vi "ODX_Read Flash Data and SA2.vi"(8 "error in":errorcluster, 11 "ODX File Path":path) -> (0 "error out":errorcluster, 1 "Download Parameter":T1, 2 "SA2 Operator":T2[](array[typedef]) {"Wert" format="%.0x"}, 3 "Flash Data Array":u8[](array[numeric]))   [LabVIEW 2018]
uses:
  Typedefs/Diagnose_SA2_Rechnenbefehl.ctl
  Typedefs/Diagnose_SA2_Operation_ENUM.ctl
  <vilib>/regexp/Match Regular Expression.xnode
panel:
  out "Block Size":u8[](array[numeric]) format="%.0x"
  out "Start Adress":u8[](array[numeric]) format="%.0x"
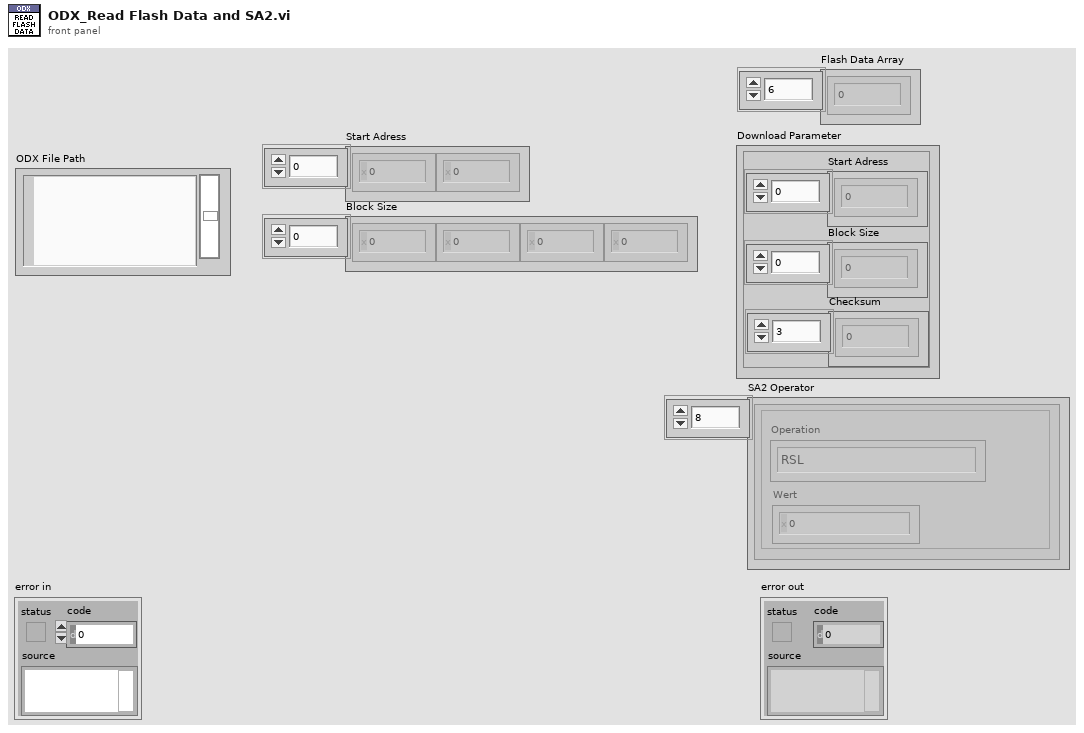
[diagram p1: front panel]
types:
  T1 = cluster{"Start Adress":u8[], "Block Size":u8[], "Checksum":u8[]}
  T2 = typedef "Diagnose_SA2_Rechnenbefehl.ctl" = cluster{"Operation":T3, "Wert":u32}
  T3 = typedef "Diagnose_SA2_Operation_ENUM.ctl" = enum16{"RSL", "RSR", "ADD", "SUB", "EOR", "Durchläufe", "NEXT", "BCC", "BRA", "Fertig"}
  T4 = enum16{"open", "replace", "create", "open or create", "replace or create", "replace or create with confirmation"}
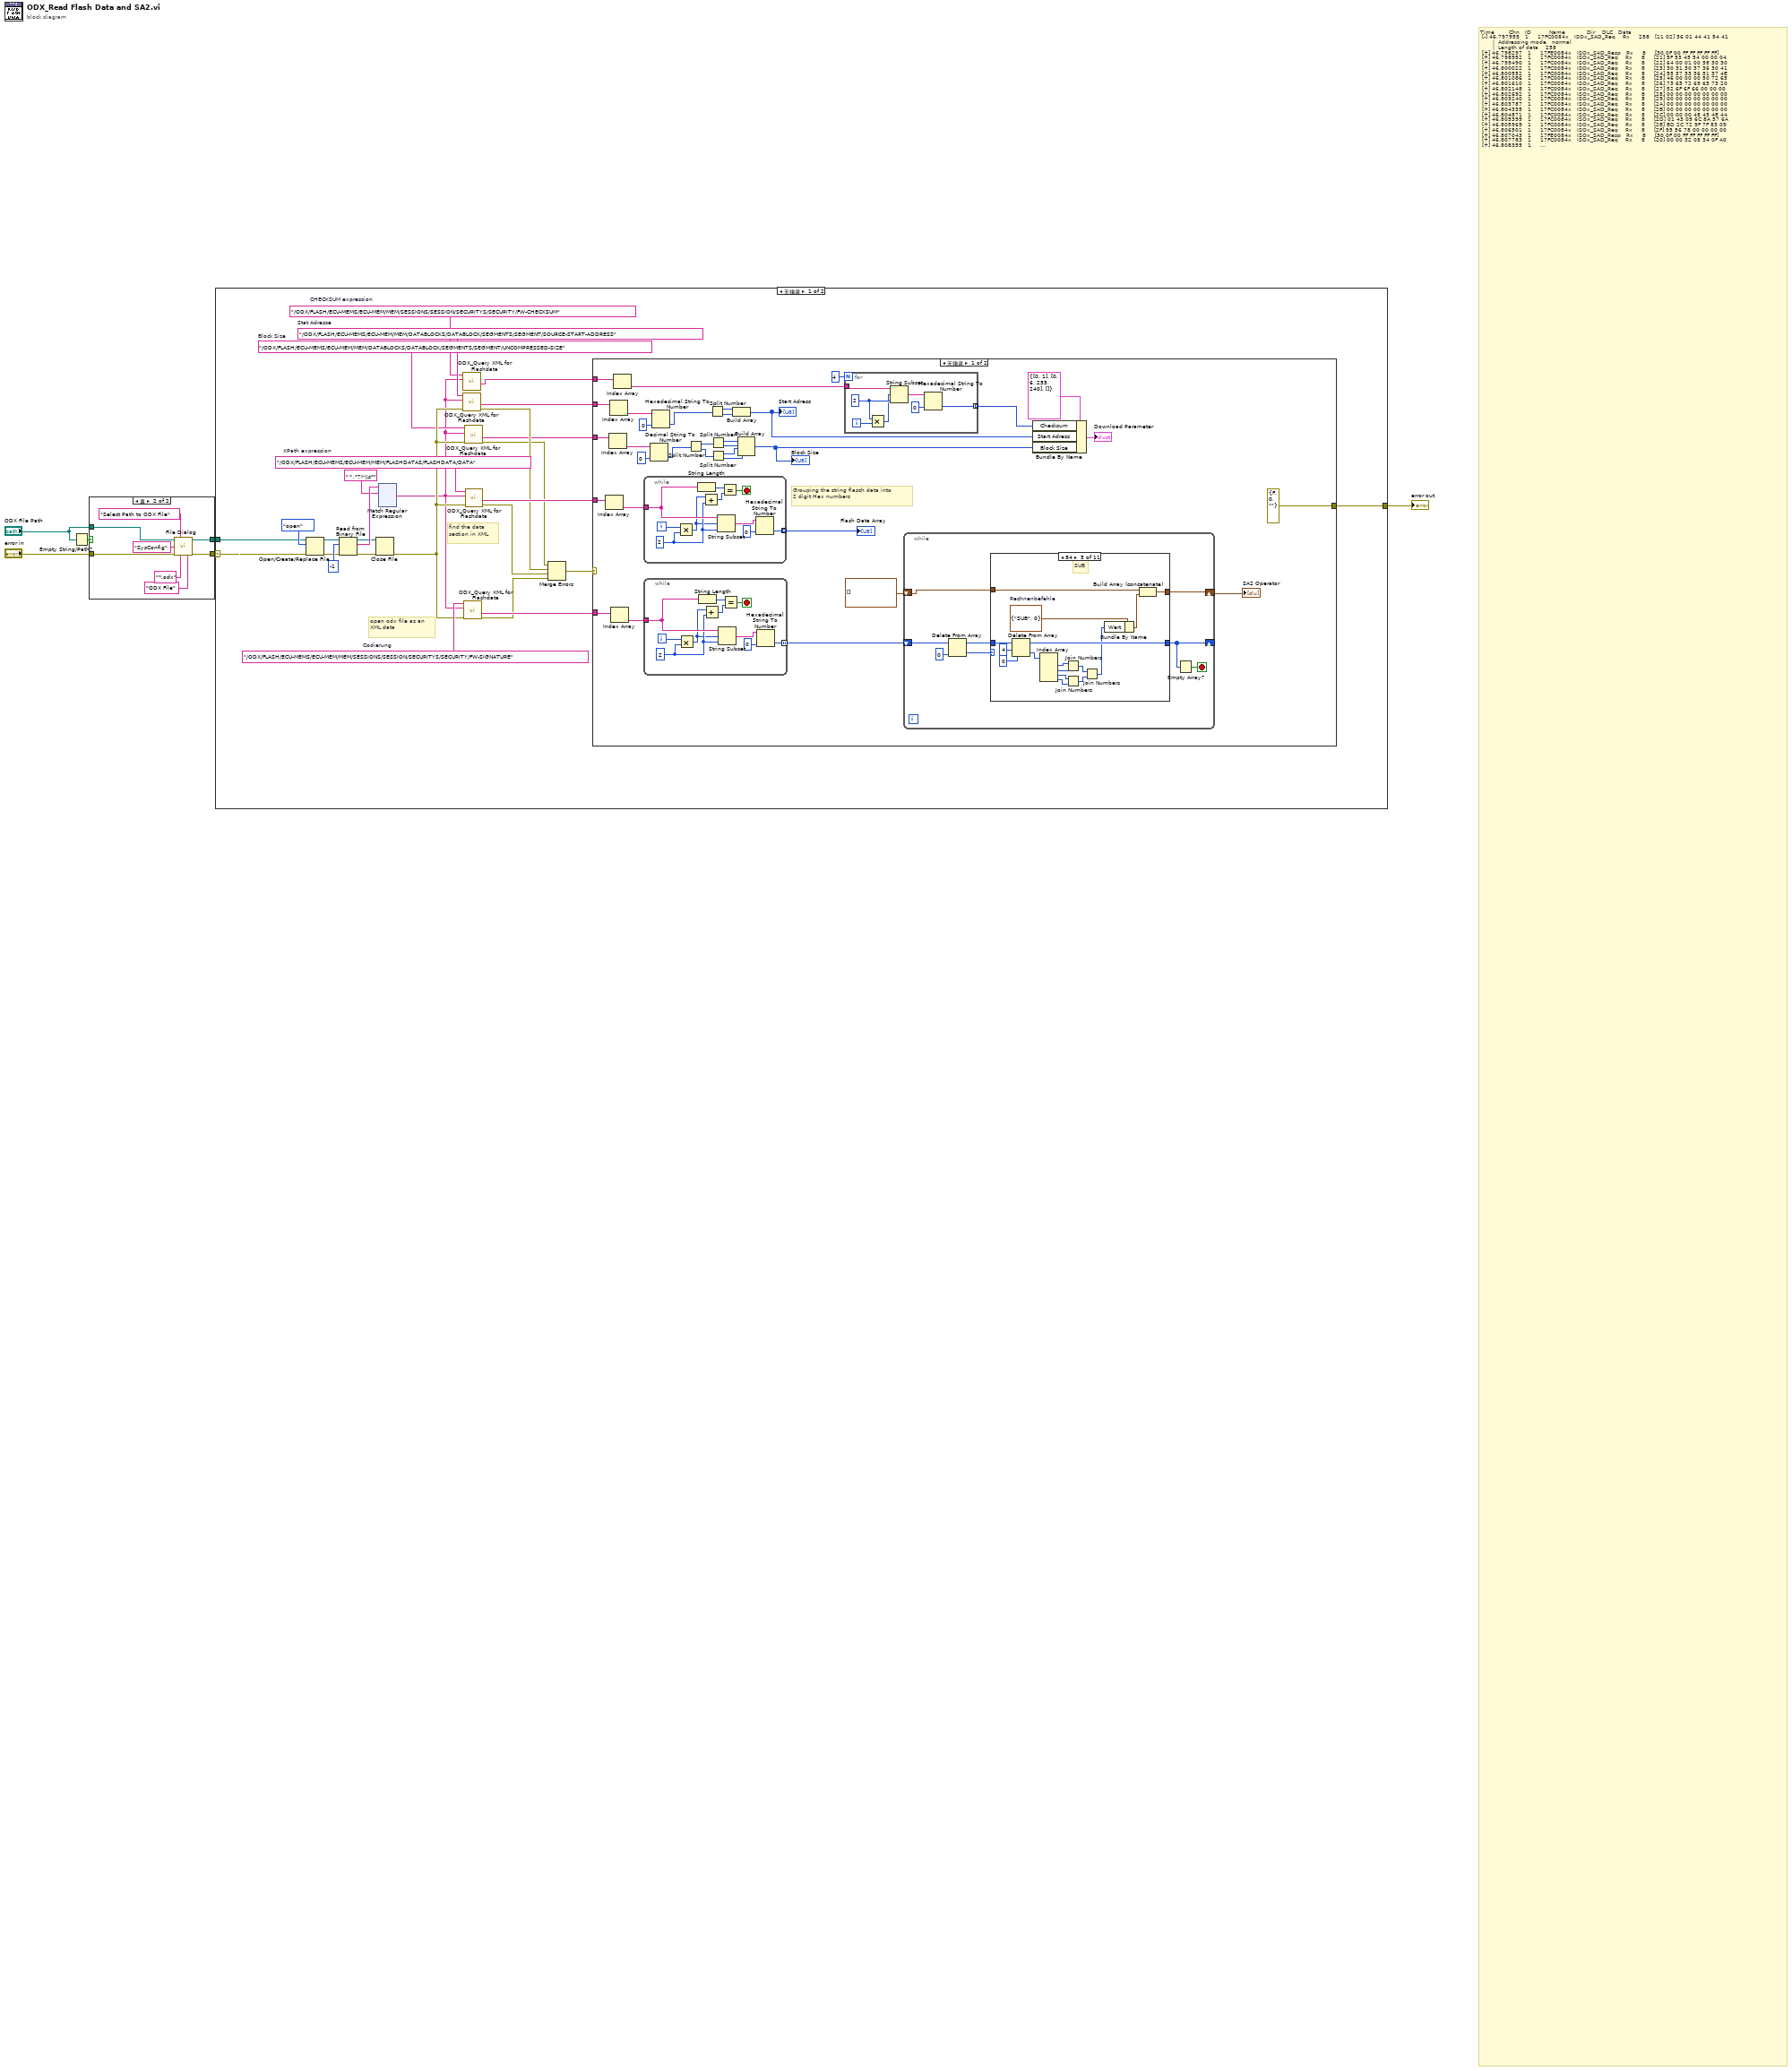
[diagram p0: block diagram]
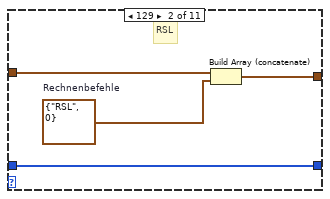
[diagram p3: hidden frame]
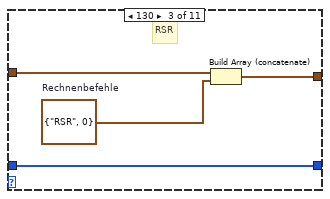
[diagram p4: hidden frame]
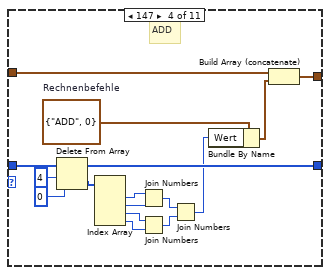
[diagram p5: hidden frame]
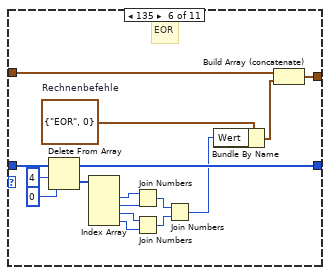
[diagram p6: hidden frame]
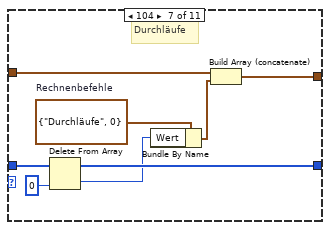
[diagram p7: hidden frame]
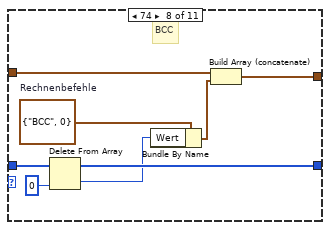
[diagram p8: hidden frame]
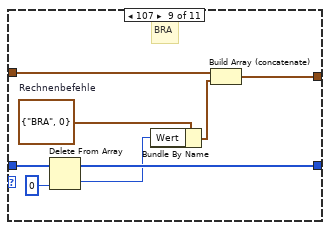
[diagram p9: hidden frame]
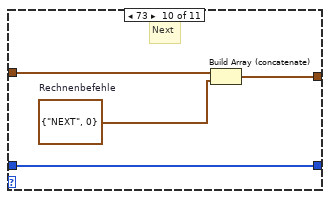
[diagram p10: hidden frame]
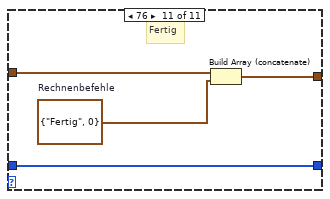
[diagram p11: hidden frame]
diagram:
  # "Time        Chn   ID          Name            Dir    DLC   Data                          \n [-] 46.797955   1     17FC0084x   ISOx_SAD_Req    Rx     258   [11 02] 36 01 44 41 54 41     \n       |  Addressing mode   normal      \n       |  Length of data    258         \n [+] 46.798297   1     17FE0084x   ISOx_SAD_Resp   Rx     8     [30 0F 00 FF FF FF FF FF]     \n [+] 46.798952   1     17FC0084x   ISOx_SAD_Req    Rx     8     [21] 5F 53 45 54 00 00 04     \n [+] 46.799490   1     17FC0084x   ISOx_SAD_Req    Rx     8     [22] 64 00 01 00 58 30 30     \n [+] 46.800022   1     17FC0084x   ISOx_SAD_Req    Rx     8     [23] 30 31 30 37 36 30 41     \n [+] 46.800552   1     17FC0084x   ISOx_SAD_Req    Rx     8     [24] 55 37 33 36 51 37 4E     \n [+] 46.801086   1     17FC0084x   ISOx_SAD_Req    Rx     8     [25] 46 00 00 00 50 72 65     \n [+] 46.801610   1     17FC0084x   ISOx_SAD_Req    Rx     8     [26] 73 65 72 69 65 73 20     \n [+] 46.802148   1     17FC0084x   ISOx_SAD_Req    Rx     8     [27] 52 6F 6F 66 00 00 00     \n [+] 46.802692   1     17FC0084x   ISOx_SAD_Req    Rx     8     [28] 00 00 00 00 00 00 00     \n [+] 46.803240   1     17FC0084x   ISOx_SAD_Req    Rx     8     [29] 00 00 00 00 00 00 00     \n [+] 46.803787   1     17FC0084x   ISOx_SAD_Req    Rx     8     [2A] 00 00 00 00 00 00 00     \n [+] 46.804335   1     17FC0084x   ISOx_SAD_Req    Rx     8     [2B] 00 00 00 00 00 00 00     \n [+] 46.804871   1     17FC0084x   ISOx_SAD_Req    Rx     8     [2C] 00 00 00 48 45 4E 44     \n [+] 46.805399   1     17FC0084x   ISOx_SAD_Req    Rx     8     [2D] 01 43 09 6C 8A 57 6A     \n [+] 46.805969   1     17FC0084x   ISOx_SAD_Req    Rx     8     [2E] BD 2C 72 9F 7F 83 09     \n [+] 46.806501   1     17FC0084x   ISOx_SAD_Req    Rx     8     [2F] 95 56 78 00 00 00 00     \n [+] 46.807043   1     17FE0084x   ISOx_SAD_Resp   Rx     8     [30 0F 00 FF FF FF FF FF]     \n [+] 46.807783   1     17FC0084x   ISOx_SAD_Req    Rx     8     [20] 00 00 32 08 34 0F A0     \n [+] 46.808355   1     17FC0084x   ISOx_SAD_Req    Rx     8     [21] 00 14 00 14 46 50 17     \n [+] 46.808930   1     17FC0084x   ISOx_SAD_Req    Rx     8     [22] 70 2E E0 1F 40 4E 20     \n [+] 46.809470   1     17FC0084x   ISOx_SAD_Req    Rx     8     [23] 1A F4 00 28 01 F4 01     \n [+] 46.810010   1     17FC0084x   ISOx_SAD_Req    Rx     8     [24] F4 00 02 00 32 00 19     \n [+] 46.810550   1     17FC0084x   ISOx_SAD_Req    Rx     8     [25] 00 96 00 32 00 00 00     \n [+] 46.811090   1     17FC0084x   ISOx_SAD_Req    Rx     8     [26] 32 00 64 00 00 00 32     \n [+] 46.811666   1     17FC0084x   ISOx_SAD_Req    Rx     8     [27] 00 64 00 50 00 50 32     \n [+] 46.812248   1     17FC0084x   ISOx_SAD_Req    Rx     8     [28] C8 01 90 07 D0 46 50     \n [+] 46.812780   1     17FC0084x   ISOx_SAD_Req    Rx     8     [29] 46 50 07 D0 6C CD 07     \n [+] 46.813316   1     17FC0084x   ISOx_SAD_Req    Rx     8     [2A] D0 1B 58 07 D0 60 00     \n [+] 46.813854   1     17FC0084x   ISOx_SAD_Req    Rx     8     [2B] 20 00 21 34 01 90 01     \n [+] 46.814389   1     17FC0084x   ISOx_SAD_Req    Rx     8     [2C] 90 01 90 01 90 01 90     \n [+] 46.814921   1     17FC0084x   ISOx_SAD_Req    Rx     8     [2D] 00 C8 5D C0 00 32 00     \n [+] 46.815459   1     17FC0084x   ISOx_SAD_Req    Rx     8     [2E] 00 01 36 06 40 00 B9     \n [+] 46.815997   1     17FE0084x   ISOx_SAD_Resp   Rx     8     [30 0F 00 FF FF FF FF FF]     \n [+] 46.816819   1     17FC0084x   ISOx_SAD_Req    Rx     8     [2F] 00 C8 00 E6 03 E8 00     \n [+] 46.817355   1     17FC0084x   ISOx_SAD_Req    Rx     8     [20] 32 00 23 00 DC 00 0A     \n [+] 46.817931   1     17FC0084x   ISOx_SAD_Req    Rx     8     [21] 00 48 1B 58 42 68 00     \n [+] 46.818466   1     17FC0084x   ISOx_SAD_Req    Rx     8     [22] C8 3E 80 3A 98 01 F4     \n [+] 46.818998   1     17FC0084x   ISOx_SAD_Req    Rx     8     [23] 2C EC 01 F4 1D 4C 03     \n [+] 46.819534   1     17FC0084x   ISOx_SAD_Req    Rx     8     [24] E8 21 34 1A 2C 02 0F     \n [+] 46.821168   1     17FE0084x   ISOx_SAD_Resp   Rx     2     [02] 76 01 [FF FF FF FF FF]   \n\n#Ende vom Block 1 (37 Messages) & Start vom Block2 (37 Messages)# \n\n[-] 46.840058   1     17FC0084x   ISOx_SAD_Req    Rx     258   [11 02] 36 02 5F 00 01 02     \n       |  Addressing mode   normal      \n       |  Length of data    258         \n [+] 46.840600   1     17FE0084x   ISOx_SAD_Resp   Rx     8     [30 0F 00 FF FF FF FF FF]     \n [+] 46.841412   1     17FC0084x   ISOx_SAD_Req    Rx     8     [21] 03 04 00 01 02 03 04     \n [+] 46.841994   1     17FC0084x   ISOx_SAD_Req    Rx     8     [22] 00 01 02 03 04 06 18     \n [+] 46.842530   1     17FC0084x   ISOx_SAD_Req    Rx     8     [23] 0A 20 1C 08 01 00 28     \n [+] 46.843066   1     17FC0084x   ISOx_SAD_Req    Rx     8     [24] 08 08 03 A0 20 C8 05     \n [+] 46.843603   1     17FC0084x   ISOx_SAD_Req    Rx     8     [25] B4 AA 05 A0 00 04 04     \n [+] 46.844129   1     17FC0084x   ISOx_SAD_Req    Rx     8     [26] 14 04 09 09 14 F6 38     \n [+] 46.844669   1     17FC0084x   ISOx_SAD_Req    Rx     8     [27] 00 00 00 01 57 C0 00     \n [+] 46.845209   1     17FC0084x   ISOx_SAD_Req    Rx     8     [28] 32 00 28 FF D8 00 14     \n [+] 46.845747   1     17FC0084x   ISOx_SAD_Req    Rx     8     [29] 07 92 00 32 00 32 01     \n [+] 46.846283   1     17FC0084x   ISOx_SAD_Req    Rx     8     [2A] 90 01 90 00 2D D8 D8     \n [+] 46.846823   1     17FC0084x   ISOx_SAD_Req    Rx     8     [2B] FF FF 0A D0 00 00 00     \n [+] 46.847361   1     17FC0084x   ISOx_SAD_Req    Rx     8     [2C] 01 57 C0 00 32 00 28     \n [+] 46.847945   1     17FC0084x   ISOx_SAD_Req    Rx     8     [2D] FF D8 00 14 0E BF 00     \n [+] 46.848480   1     17FC0084x   ISOx_SAD_Req    Rx     8     [2E] 32 00 32 01 90 01 90     \n [+] 46.849014   1     17FC0084x   ISOx_SAD_Req    Rx     8     [2F] 00 2D D8 D8 FF FF 0A     \n [+] 46.849556   1     17FE0084x   ISOx_SAD_Resp   Rx     8     [30 0F 00 FF FF FF FF FF]     \n [+] 46.850360   1     17FC0084x   ISOx_SAD_Req    Rx     8     [20] D0 00 00 01 24 60 FA     \n [+] 46.850894   1     17FC0084x   ISOx_SAD_Req    Rx     8     [21] 08 E3 12 C1 5F A2 47     \n [+] 46.851422   1     17FC0084x   ISOx_SAD_Req    Rx     8     [22] 95 E4 7E E2 BF BD 00     \n [+] 46.851964   1     17FC0084x   ISOx_SAD_Req    Rx     8     [23] 00 00 00 00 32 32 00     \n [+] 46.852510   1     17FC0084x   ISOx_SAD_Req    Rx     8     [24] 00 00 00 00 00 00 00     \n [+] 46.853051   1     17FC0084x   ISOx_SAD_Req    Rx     8     [25] 00 00 00 00 32 32 00     \n [+] 46.853643   1     17FC0084x   ISOx_SAD_Req    Rx     8     [26] 00 00 00 00 00 00 00     \n [+] 46.854183   1     17FC0084x   ISOx_SAD_Req    Rx     8     [27] 00 00 00 00 32 32 00     \n [+] 46.854729   1     17FC0084x   ISOx_SAD_Req    Rx     8     [28] 00 00 00 00 00 00 00     \n [+] 46.855269   1     17FC0084x   ISOx_SAD_Req    Rx     8     [29] 00 00 00 00 32 32 00     \n [+] 46.855811   1     17FC0084x   ISOx_SAD_Req    Rx     8     [2A] 00 00 00 00 00 00 00     \n [+] 46.856347   1     17FC0084x   ISOx_SAD_Req    Rx     8     [2B] 00 00 00 00 32 32 00     \n [+] 46.856899   1     17FC0084x   ISOx_SAD_Req    Rx     8     [2C] 00 00 00 00 00 00 00     \n [+] 46.857435   1     17FC0084x   ISOx_SAD_Req    Rx     8     [2D] 00 00 00 00 32 32 00     \n [+] 46.857984   1     17FC0084x   ISOx_SAD_Req    Rx     8     [2E] 00 00 00 00 00 00 00     \n [+] 46.858524   1     17FE0084x   ISOx_SAD_Resp   Rx     8     [30 0F 00 FF FF FF FF FF]     \n [+] 46.859390   1     17FC0084x   ISOx_SAD_Req    Rx     8     [2F] 00 00 00 00 32 32 00     \n [+] 46.859936   1     17FC0084x   ISOx_SAD_Req    Rx     8     [20] 00 00 00 00 00 00 00     \n [+] 46.860474   1     17FC0084x   ISOx_SAD_Req    Rx     8     [21] 00 32 06 A4 00 C8 00     \n [+] 46.861014   1     17FC0084x   ISOx_SAD_Req    Rx     8     [22] C8 00 14 03 20 0F A0     \n [+] 46.861550   1     17FC0084x   ISOx_SAD_Req    Rx     8     [23] 00 00 00 F0 07 08 00     \n [+] 46.862084   1     17FC0084x   ISOx_SAD_Req    Rx     8     [24] 32 00 F0 75 30 00 00     \n [+] 46.863713   1     17FE0084x   ISOx_SAD_Resp   Rx     2     [02] 76 02 [FF FF FF FF FF]   \n\n#Ende vom Block 2 (37 Messages) & Start vom Block 3 (37 Messages)# \n\n [-] 46.886746   1     17FC0084x   ISOx_SAD_Req    Rx     258   [11 02] 36 03 00 00 3A 98     \n       |  Addressing mode   normal      \n       |  Length of data    258         \n [+] 46.887288   1     17FE0084x   ISOx_SAD_Resp   Rx     8     [30 0F 00 FF FF FF FF FF]     \n [+] 46.888093   1     17FC0084x   ISOx_SAD_Req    Rx     8     [21] 2A F8 01 48 01 48 0B     \n [+] 46.888629   1     17FC0084x   ISOx_SAD_Req    Rx     8     [22] B8 07 08 00 F0 00 F0     \n [+] 46.889165   1     17FC0084x   ISOx_SAD_Req    Rx     8     [23] 00 32 32 C8 00 00 00     \n [+] 46.889703   1     17FC0084x   ISOx_SAD_Req    Rx     8     [24] 50 80 00 3E 80 0C CD     \n [+] 46.890233   1     17FC0084x   ISOx_SAD_Req    Rx     8     [25] 17 70 F3 33 00 00 17     \n [+] 46.890771   1     17FC0084x   ISOx_SAD_Req    Rx     8     [26] 70 00 7D 00 32 00 32     \n [+] 46.891353   1     17FC0084x   ISOx_SAD_Req    Rx     8     [27] 00 7D 00 64 02 00 00     \n [+] 46.891892   1     17FC0084x   ISOx_SAD_Req    Rx     8     [28] 80 0E 10 0C 80 3E 80     \n [+] 46.892434   1     17FC0084x   ISOx_SAD_Req    Rx     8     [29] 01 04 01 01 04 02 03     \n [+] 46.892972   1     17FC0084x   ISOx_SAD_Req    Rx     8     [2A] 03 03 08 08 B4 00 04     \n [+] 46.893504   1     17FC0084x   ISOx_SAD_Req    Rx     8     [2B] 14 FF 02 00 00 22 FD     \n [+] 46.894034   1     17FC0084x   ISOx_SAD_Req    Rx     8     [2C] 19 14 C8 06 00 14 08     \n [+] 46.894574   1     17FC0084x   ISOx_SAD_Req    Rx     8     [2D] 00 0A 3C 41 32 41 5F     \n [+] 46.895106   1     17FC0084x   ISOx_SAD_Req    Rx     8     [2E] 04 32 14 08 28 05 14     \n [+] 46.895646   1     17FC0084x   ISOx_SAD_Req    Rx     8     [2F] 00 64 50 3C 1E 1E 19     \n [+] 46.896186   1     17FE0084x   ISOx_SAD_Resp   Rx     8     [30 0F 00 FF FF FF FF FF]     \n [+] 46.897043   1     17FC0084x   ISOx_SAD_Req    Rx     8     [20] 1E 19 01 37 00 00 00     \n [+] 46.897575   1     17FC0084x   ISOx_SAD_Req    Rx     8     [21] 02 C8 00 0A 14 0C 21     \n [+] 46.898107   1     17FC0084x   ISOx_SAD_Req    Rx     8     [22] 21 0B 32 00 05 08 10     \n [+] 46.898647   1     17FC0084x   ISOx_SAD_Req    Rx     8     [23] E7 28 04 01 01 00 01     \n [+] 46.899180   1     17FC0084x   ISOx_SAD_Req    Rx     8     [24] 02 01 04 64 FF FF 1E     \n [+] 46.899713   1     17FC0084x   ISOx_SAD_Req    Rx     8     [25] 02 0A 28 01 74 4B 00     \n [+] 46.900247   1     17FC0084x   ISOx_SAD_Req    Rx     8     [26] 28 02 87 2D 01 0A 06     \n [+] 46.900781   1     17FC0084x   ISOx_SAD_Req    Rx     8     [27] 02 BC 00 32 0D AC 01     \n [+] 46.901317   1     17FC0084x   ISOx_SAD_Req    Rx     8     [28] A9 01 A9 00 14 03 20     \n [+] 46.901858   1     17FC0084x   ISOx_SAD_Req    Rx     8     [29] 0F A0 00 00 00 32 0E     \n [+] 46.902400   1     17FC0084x   ISOx_SAD_Req    Rx     8     [2A] 10 00 00 00 00 75 30     \n [+] 46.902984   1     17FC0084x   ISOx_SAD_Req    Rx     8     [2B] 00 00 00 00 3A 98 2A     \n [+] 46.903518   1     17FC0084x   ISOx_SAD_Req    Rx     8     [2C] F8 01 48 01 48 0B B8     \n [+] 46.904061   1     17FC0084x   ISOx_SAD_Req    Rx     8     [2D] 0E 10 00 64 00 00 00     \n [+] 46.904605   1     17FC0084x   ISOx_SAD_Req    Rx     8     [2E] 00 32 C8 00 00 00 50     \n [+] 46.905141   1     17FE0084x   ISOx_SAD_Resp   Rx     8     [30 0F 00 FF FF FF FF FF]     \n [+] 46.905951   1     17FC0084x   ISOx_SAD_Req    Rx     8     [2F] 80 00 FF FF 0C CD 17     \n [+] 46.906482   1     17FC0084x   ISOx_SAD_Req    Rx     8     [20] 70 F3 33 00 00 0B B8     \n [+] 46.907025   1     17FC0084x   ISOx_SAD_Req    Rx     8     [21] 00 7D 00 32 00 32 00     \n [+] 46.907563   1     17FC0084x   ISOx_SAD_Req    Rx     8     [22] 7D 00 64 02 00 00 80     \n [+] 46.908099   1     17FC0084x   ISOx_SAD_Req    Rx     8     [23] 0E 10 0C 80 3E 80 01     \n [+] 46.908637   1     17FC0084x   ISOx_SAD_Req    Rx     8     [24] 04 01 01 04 02 03 03     \n [+] 46.910288   1     17FE0084x   ISOx_SAD_Resp   Rx     2     [02] 76 03 [FF FF FF FF FF]   \n\n#Ende vom Block 3 (37 Messages) & Start vom Block 4 (37 Messages)# \n\n [-] 46.922703   1     17FC0084x   ISOx_SAD_Req    Rx     258   [11 02] 36 04 03 08 08 AB     \n       |  Addressing mode   normal      \n       |  Length of data    258         \n [+] 46.923243   1     17FE0084x   ISOx_SAD_Resp   Rx     8     [30 0F 00 FF FF FF FF FF]     \n [+] 46.924019   1     17FC0084x   ISOx_SAD_Req    Rx     8     [21] 01 04 14 FF 02 00 00     \n [+] 46.924593   1     17FC0084x   ISOx_SAD_Req    Rx     8     [22] 22 FD 19 14 C8 14 1E     \n [+] 46.925135   1     17FC0084x   ISOx_SAD_Req    Rx     8     [23] 00 00 00 0A 3C 3C 00     \n [+] 46.925673   1     17FC0084x   ISOx_SAD_Req    Rx     8     [24] 00 5F 04 32 14 08 08     \n [+] 46.926215   1     17FC0084x   ISOx_SAD_Req    Rx     8     [25] 00 00 00 00 50 3C 1E     \n [+] 46.926749   1     17FC0084x   ISOx_SAD_Req    Rx     8     [26] 1E 00 00 23 01 3D 00     \n [+] 46.927330   1     17FC0084x   ISOx_SAD_Req    Rx     8     [27] 00 00 02 C8 00 0A 14     \n [+] 46.927906   1     17FC0084x   ISOx_SAD_Req    Rx     8     [28] 05 21 21 0B 32 00 05     \n [+] 46.928438   1     17FC0084x   ISOx_SAD_Req    Rx     8     [29] 08 10 E7 28 04 01 01     \n [+] 46.928978   1     17FC0084x   ISOx_SAD_Req    Rx     8     [2A] 00 01 02 01 04 64 FF     \n [+] 46.929518   1     17FC0084x   ISOx_SAD_Req    Rx     8     [2B] FF 1E 02 0A 28 01 74     \n [+] 46.930046   1     17FC0084x   ISOx_SAD_Req    Rx     8     [2C] 4B 00 28 02 87 2D 01     \n [+] 46.930580   1     17FC0084x   ISOx_SAD_Req    Rx     8     [2D] 0A 06 02 BC 00 00 00     \n [+] 46.931128   1     17FC0084x   ISOx_SAD_Req    Rx     8     [2E] 00 00 00 00 00 00 00     \n [+] 46.931673   1     17FC0084x   ISOx_SAD_Req    Rx     8     [2F] 00 00 00 00 00 00 00     \n [+] 46.932215   1     17FE0084x   ISOx_SAD_Resp   Rx     8     [30 0F 00 FF FF FF FF FF]     \n [+] 46.933035   1     17FC0084x   ISOx_SAD_Req    Rx     8     [20] 00 00 00 00 00 00 00     \n [+] 46.933625   1     17FC0084x   ISOx_SAD_Req    Rx     8     [21] 00 00 00 00 00 00 00     \n [+] 46.934170   1     17FC0084x   ISOx_SAD_Req    Rx     8     [22] 00 00 00 00 00 00 00     \n [+] 46.934716   1     17FC0084x   ISOx_SAD_Req    Rx     8     [23] 00 00 00 00 00 00 00     \n [+] 46.935264   1     17FC0084x   ISOx_SAD_Req    Rx     8     [24] 00 00 00 00 00 00 00     \n [+] 46.935806   1     17FC0084x   ISOx_SAD_Req    Rx     8     [25] 00 00 00 00 00 00 00     \n [+] 46.936350   1     17FC0084x   ISOx_SAD_Req    Rx     8     [26] 00 00 00 00 00 00 00     \n [+] 46.936902   1     17FC0084x   ISOx_SAD_Req    Rx     8     [27] 00 00 00 00 00 00 00     \n [+] 46.937446   1     17FC0084x   ISOx_SAD_Req    Rx     8     [28] 00 00 00 00 00 00 00     \n [+] 46.937994   1     17FC0084x   ISOx_SAD_Req    Rx     8     [29] 00 00 00 00 00 00 00     \n [+] 46.938541   1     17FC0084x   ISOx_SAD_Req    Rx     8     [2A] 00 00 00 00 00 00 00     \n [+] 46.939089   1     17FC0084x   ISOx_SAD_Req    Rx     8     [2B] 00 00 00 00 00 00 00     \n [+] 46.939683   1     17FC0084x   ISOx_SAD_Req    Rx     8     [2C] 00 00 00 00 00 00 00     \n [+] 46.940227   1     17FC0084x   ISOx_SAD_Req    Rx     8     [2D] 00 00 00 00 00 00 00     \n [+] 46.940773   1     17FC0084x   ISOx_SAD_Req    Rx     8     [2E] 00 00 00 00 00 00 00     \n [+] 46.941315   1     17FE0084x   ISOx_SAD_Resp   Rx     8     [30 0F 00 FF FF FF FF FF]     \n [+] 46.942125   1     17FC0084x   ISOx_SAD_Req    Rx     8     [2F] 00 00 00 00 00 00 00     \n [+] 46.942675   1     17FC0084x   ISOx_SAD_Req    Rx     8     [20] 00 00 00 00 00 00 00     \n [+] 46.943219   1     17FC0084x   ISOx_SAD_Req    Rx     8     [21] 00 00 00 00 00 00 00     \n [+] 46.943768   1     17FC0084x   ISOx_SAD_Req    Rx     8     [22] 00 00 00 00 00 00 00     \n [+] 46.944314   1     17FC0084x   ISOx_SAD_Req    Rx     8     [23] 00 00 00 00 00 00 00     \n [+] 46.944860   1     17FC0084x   ISOx_SAD_Req    Rx     8     [24] 00 00 00 00 00 00 00     \n [+] 46.946525   1     17FE0084x   ISOx_SAD_Resp   Rx     2     [02] 76 04 [FF FF FF FF FF]   \n\n#Ende vom Block 4 (37 Messages) & Start vom Block 5 (37 Messages)# \n\n [-] 46.958341   1     17FC0084x   ISOx_SAD_Req    Rx     106   [10 6A] 36 05 00 00 00 00     \n       |  Addressing mode   normal      \n       |  Length of data    106         \n [+] 46.958861   1     17FE0084x   ISOx_SAD_Resp   Rx     8     [30 0F 00 FF FF FF FF FF]     \n [+] 46.959681   1     17FC0084x   ISOx_SAD_Req    Rx     8     [21] 00 00 00 00 00 00 00     \n [+] 46.960151   1     17FC0084x   ISOx_SAD_Req    Rx     8     [22] 00 00 00 00 00 00 00     \n [+] 46.960735   1     17FC0084x   ISOx_SAD_Req    Rx     8     [23] 00 00 00 00 00 00 00     \n [+] 46.961321   1     17FC0084x   ISOx_SAD_Req    Rx     8     [24] 00 00 00 00 00 00 00     \n [+] 46.961869   1     17FC0084x   ISOx_SAD_Req    Rx     8     [25] 00 00 00 00 00 00 00     \n [+] 46.962419   1     17FC0084x   ISOx_SAD_Req    Rx     8     [26] 00 00 00 00 00 00 00     \n [+] 46.962970   1     17FC0084x   ISOx_SAD_Req    Rx     8     [27] 00 00 00 00 00 00 00     \n [+] 46.963516   1     17FC0084x   ISOx_SAD_Req    Rx     8     [28] 00 00 00 00 00 00 00     \n [+] 46.964102   1     17FC0084x   ISOx_SAD_Req    Rx     8     [29] 00 00 00 00 00 00 00     \n [+] 46.964648   1     17FC0084x   ISOx_SAD_Req    Rx     8     [2A] 00 00 00 00 00 00 00     \n [+] 46.965196   1     17FC0084x   ISOx_SAD_Req    Rx     8     [2B] 00 00 00 00 00 00 00     \n [+] 46.965786   1     17FC0084x   ISOx_SAD_Req    Rx     8     [2C] 00 00 00 00 00 00 00     \n [+] 46.966294   1     17FC0084x   ISOx_SAD_Req    Rx     8     [2D] 98 56 B2 A9 44 41 54     \n [+] 46.966830   1     17FC0084x   ISOx_SAD_Req    Rx     8     [2E] 41 5F 45 4E 44 FF FF     \n [+] 46.967362   1     17FC0084x   ISOx_SAD_Req    Rx     8     [2F] FF FF 55 55 55 55 55    \n\n#Ende Flaschen; Beenden mit 0x55 wenn keine Daten vorhandeln#\n \n [+] 46.968451   1     17FE0084x   ISOx_SAD_Resp   Rx     2     [02] 76 05 [FF FF FF FF FF]"
  n1 = Empty String/Path?(string/path="ODX File Path") -> (empty?=w6:bool)
  n2 = case shown="真" w6 {
    tunnel: "error in" -> [w8 w16]
    tunnel: [w7 w11] -> w3
    tunnel: [w8 w10] -> w1
    tunnel: "ODX File Path" -> [w7 w9]
    frame False {
    }
    frame True {
      n3 = call "File Dialog"("start path"=w9, "prompt"="Select Path to ODX File" ("Prompt"), "default name"="SysConfig", "error in"=w16, "pattern (all files)"="*.odx" ("pattern"), "pattern label"="ODX File") -> ("selected path"=w11:path, "error out"=w10:errorcluster)  [unwired: 6 in, 2 out]
    }
  }
  n4 = case shown="无错误" w1 {
    selector: w1 -> [w27 w315]
    tunnel: w3 -> [w29 _]
    tunnel: [w28 w315] -> w2
    frame No Error {
      w18 = "/ODX/FLASH/ECU-MEMS/ECU-MEM/MEM/SESSIONS/SESSION/SECURITYS/SECURITY/FW-CHECKSUM"  # CHECKSUM expression
      w22 = "/ODX/FLASH/ECU-MEMS/ECU-MEM/MEM/DATABLOCKS/DATABLOCK/SEGMENTS/SEGMENT/UNCOMPRESSED-SIZE"  # Block Size
      w26 = "/ODX/FLASH/ECU-MEMS/ECU-MEM/MEM/DATABLOCKS/DATABLOCK/SEGMENTS/SEGMENT/SOURCE-START-ADDRESS"  # Stat Adresse
      w41 = "/ODX/FLASH/ECU-MEMS/ECU-MEM/MEM/SESSIONS/SESSION/SECURITYS/SECURITY/FW-SIGNATURE"  # Codierung
      w44 = "/ODX/FLASH/ECU-MEMS/ECU-MEM/MEM/FLASHDATAS/FLASHDATA/DATA"  # XPath expression
      # "find the data\nsection in XML"
      # "open odx file as an\nXML data"
      n5 = Open/Create/Replace File(file path (use dialog)=w29, error in=w27, operation (0:open)=T4."open") -> (refnum out=w32:refnum<file>, error out=w33:errorcluster)  [unwired: 3 in, 1 out]
      n6 = Read from Binary File(8:w33, 10:-1 ("count (1)"), 11:w32) -> (0:w31:errorcluster, 2:w37:string, 3:w30:refnum<file>)  [unwired: 3 in, 1 out]
      n7 = Close File(refnum=w30, error in=w31) -> (error out=w23:errorcluster)  [unwired: 1 out]
      n8 = xnode "Match Regular Expression"("input string"=w37, "regular expression"="^.*?>\\s*") -> ("after match"=w19:string)  [unwired: 4 in, 4 out]
      n9 = call "ODX_Query XML for Flashdata.vi"("XML document"=w19, "XPath expression"=w18) -> ("Result Array"=w17:string[])  [unwired: 8 in, 1 out]
      n10 = call "ODX_Query XML for Flashdata.vi"("error in (no error)"=w23, "XML document"=w19, "XPath expression"=w26) -> ("error out"=w25:errorcluster, "Result Array"=w24:string[])  [unwired: 7 in]
      n11 = call "ODX_Query XML for Flashdata.vi"("error in (no error)"=w23, "XML document"=w19, "XPath expression"=w41) -> ("error out"=w38:errorcluster, "Result Array"=w40:string[])  [unwired: 7 in]
      n12 = call "ODX_Query XML for Flashdata.vi"("error in (no error)"=w23, "XML document"=w19, "XPath expression"=w22) -> ("error out"=w21:errorcluster, "Result Array"=w20:string[])  [unwired: 7 in]
      n13 = call "ODX_Query XML for Flashdata.vi"("error in (no error)"=w23, "XML document"=w19, "XPath expression"=w44) -> ("error out"=w42:errorcluster, "Result Array"=w43:string[])  [unwired: 7 in]
      n14 = Merge Errors(w21, w25, w42, w38) -> (w39:errorcluster)
      n15 = case shown="无错误" w39 {
        selector: w39 -> [_ w314]
        tunnel: w43 -> [w188 _]
        tunnel: [errorcluster {"status"=FALSE, "code"=0, "source"=""} ("error IO") w314] -> w28
        tunnel: w40 -> [w183 _]
        tunnel: w24 -> [w179 _]
        tunnel: w20 -> [w175 _]
        tunnel: w17 -> [w159 _]
        frame No Error {
          # "Grouping the string flasch data into\n2 digit Hex numbers"
          n16 = Index Array(array=w188) -> (element=w187:string)  [unwired: 1 in]
          n17 = Index Array(array=w175) -> (element=w174:string)  [unwired: 1 in]
          n18 = Index Array(array=w179) -> (element=w178:string)  [unwired: 1 in]
          n19 = Index Array(array=w183) -> (element=w184:string)  [unwired: 1 in]
          n20 = Index Array(array=w159) -> (element=w157:string)  [unwired: 1 in]
          n21 = while {
            tunnel: w187 -> [w312]
            tunnel: [w304] -> w186 mode=indexing
            i -> [w313]
            stop <- w309 stop-if-true
            w311 = 2 ("length (rest)")
            n22 = Multiply(x=w313, y=w311) -> (x*y=w310:i32)
            n23 = String Length(string=w312) -> (length=w308:i32)
            n24 = Add(x=w310, y=w311) -> (x+y=w307:i32)
            n25 = String Subset(string=w312, offset (0)=w310, length (rest)=w311) -> (substring=w306:string)
            n26 = Equal?(x=w308, y=w307) -> (x = y?=w309:bool)
            n27 = Hexadecimal String To Number(string=w306, default (0uL)=u8 0 ("default (0 U32)")) -> (number=w304:u8)  [unwired: 1 in, 1 out]
          }
          "Flash Data Array" <- w186
          n28 = while {
            tunnel: w184 -> [w302]
            tunnel: [w294] -> w182 mode=indexing
            i -> [w303]
            stop <- w299 stop-if-true
            w301 = 2 ("length (rest)")
            n29 = Multiply(x=w303, y=w301) -> (x*y=w300:i32)
            n30 = String Length(string=w302) -> (length=w298:i32)
            n31 = Add(x=w300, y=w301) -> (x+y=w297:i32)
            n32 = String Subset(string=w302, offset (0)=w300, length (rest)=w301) -> (substring=w296:string)
            n33 = Equal?(x=w298, y=w297) -> (x = y?=w299:bool)
            n34 = Hexadecimal String To Number(string=w296, default (0uL)=u8 0 ("default (0 U32)")) -> (number=w294:u8)  [unwired: 1 in, 1 out]
          }
          n35 = Decimal String To Number(string=w174, default (0L)=u32 0 ("default (0 I32)")) -> (number=w173:u32)  [unwired: 1 in, 1 out]
          n36 = Hexadecimal String To Number(string=w178, default (0uL)=u16 0 ("default (0 U32)")) -> (number=w177:u16)  [unwired: 1 in, 1 out]
          n37 = Split Number(x=w173) -> (hi(x)=w172:u16, lo(x)=w171:u16)
          n38 = Split Number(x=w177) -> (hi(x)=w170:u8, lo(x)=w169:u8)
          n39 = Split Number(x=w172) -> (hi(x)=w168:u8, lo(x)=w167:u8)
          n40 = Split Number(x=w171) -> (hi(x)=w166:u8, lo(x)=w165:u8)
          n41 = Build Array(w170, w169) -> (w162:u8[])
          "Start Adress" <- w162
          n42 = Build Array(w168, w167, w166, w165) -> (w161:u8[])
          "Block Size" <- w161
          n43 = for {
            N: 4 -> [_]
            tunnel: w157 -> [w195]
            tunnel: [w189] -> w156 mode=indexing
            i -> [w194]
            w193 = 2 ("length (rest)")
            n44 = Multiply(x=w193, y=w194) -> (x*y=w192:i32)
            n45 = String Subset(string=w195, offset (0)=w192, length (rest)=w193) -> (substring=w191:string)
            n46 = Hexadecimal String To Number(string=w191, default (0uL)=u8 0 ("default (0 I32)")) -> (number=w189:u8)  [unwired: 1 in, 1 out]
          }
          n47 = while {
            shift-right: [w197] -> _
            shift-left: w182 -> [w203]
            shift-right: [w199] -> w180
            shift-left: T2[] [] -> [w198]
            stop <- w196 stop-if-true
            n48 = Delete From Array(array=w203, index=0) -> (deleted portion=w201:u8, array with subset deleted=w200:u8[])  [unwired: 1 in]
            n49 = case shown="84" w201 {
              tunnel: w200 -> [w204 w209 w213 w227 w243 w259 w267 w275 w283 w286 w290]
              tunnel: [w204 w209 w213 w224 w240 w256 w265 w273 w281 w286 w290] -> w197
              tunnel: [w205 w207 w211 w229 w245 w261 w269 w277 w285 w289 w293] -> w199
              tunnel: w198 -> [w205 w206 w210 w228 w244 w260 w268 w276 w284 w288 w292]
              frame 0, Default {
              }
              frame 129 {
                w208 = T2 {"Operation"=enum."RSL", "Wert"=0}  # Rechnenbefehle
                # "RSL"
                n50 = Build Array (concatenate)(w206, w208) -> (w207:T2[])
              }
              frame 130 {
                w212 = T2 {"Operation"=enum."RSR", "Wert"=0}  # Rechnenbefehle
                # "RSR"
                n51 = Build Array (concatenate)(w210, w212) -> (w211:T2[])
              }
              frame 147 {
                w223 = T2 {"Operation"=enum."ADD", "Wert"=0}  # Rechnenbefehle
                # "ADD"
                n52 = Delete From Array(array=w227, length=4, index=0) -> (deleted portion=w221:u8[], array with subset deleted=w224:u8[])
                n53 = Index Array(array=w221) -> (element #1=w220:u8, element #2=w219:u8, element #3=w218:u8, element #4=w217:u8)  [unwired: 4 in]
                n54 = Join Numbers(hi=w220, lo=w219) -> ((hi.lo)=w216:u16)
                n55 = Join Numbers(hi=w218, lo=w217) -> ((hi.lo)=w215:u16)
                n56 = Join Numbers(hi=w216, lo=w215) -> ((hi.lo)=w214:u32)
                n57 = Bundle By Name(cluster=w223, "Wert"=w214) -> (w222:T2)
                n58 = Build Array (concatenate)(w228, w222) -> (w229:T2[])
              }
              frame 132 {
                w239 = T2 {"Operation"=enum."SUB", "Wert"=0}  # Rechnenbefehle
                # "SUB"
                n59 = Delete From Array(array=w243, length=4, index=0) -> (deleted portion=w231:u8[], array with subset deleted=w240:u8[])
                n60 = Index Array(array=w231) -> (element #1=w237:u8, element #2=w236:u8, element #3=w235:u8, element #4=w234:u8)  [unwired: 4 in]
                n61 = Join Numbers(hi=w237, lo=w236) -> ((hi.lo)=w233:u16)
                n62 = Join Numbers(hi=w235, lo=w234) -> ((hi.lo)=w232:u16)
                n63 = Join Numbers(hi=w233, lo=w232) -> ((hi.lo)=w230:u32)
                n64 = Bundle By Name(cluster=w239, "Wert"=w230) -> (w238:T2)
                n65 = Build Array (concatenate)(w244, w238) -> (w245:T2[])
              }
              frame 135 {
                w255 = T2 {"Operation"=enum."EOR", "Wert"=0}  # Rechnenbefehle
                # "EOR"
                n66 = Delete From Array(array=w259, length=4, index=0) -> (deleted portion=w247:u8[], array with subset deleted=w256:u8[])
                n67 = Index Array(array=w247) -> (element #1=w253:u8, element #2=w252:u8, element #3=w251:u8, element #4=w250:u8)  [unwired: 4 in]
                n68 = Join Numbers(hi=w253, lo=w252) -> ((hi.lo)=w249:u16)
                n69 = Join Numbers(hi=w251, lo=w250) -> ((hi.lo)=w248:u16)
                n70 = Join Numbers(hi=w249, lo=w248) -> ((hi.lo)=w246:u32)
                n71 = Bundle By Name(cluster=w255, "Wert"=w246) -> (w254:T2)
                n72 = Build Array (concatenate)(w260, w254) -> (w261:T2[])
              }
              frame 104 {
                w264 = T2 {"Operation"=enum."Durchläufe", "Wert"=0}  # Rechnenbefehle
                # "Durchläufe"
                n73 = Delete From Array(array=w267, index=0) -> (deleted portion=w262:u8, array with subset deleted=w265:u8[])  [unwired: 1 in]
                n74 = Bundle By Name(cluster=w264, "Wert"=w262) -> (w263:T2)
                n75 = Build Array (concatenate)(w268, w263) -> (w269:T2[])
              }
              frame 74 {
                w272 = T2 {"Operation"=enum."BCC", "Wert"=0}  # Rechnenbefehle
                # "BCC"
                n76 = Delete From Array(array=w275, index=0) -> (deleted portion=w270:u8, array with subset deleted=w273:u8[])  [unwired: 1 in]
                n77 = Bundle By Name(cluster=w272, "Wert"=w270) -> (w271:T2)
                n78 = Build Array (concatenate)(w276, w271) -> (w277:T2[])
              }
              frame 107 {
                w280 = T2 {"Operation"=enum."BRA", "Wert"=0}  # Rechnenbefehle
                # "BRA"
                n79 = Delete From Array(array=w283, index=0) -> (deleted portion=w278:u8, array with subset deleted=w281:u8[])  [unwired: 1 in]
                n80 = Bundle By Name(cluster=w280, "Wert"=w278) -> (w279:T2)
                n81 = Build Array (concatenate)(w284, w279) -> (w285:T2[])
              }
              frame 73 {
                w287 = T2 {"Operation"=enum."NEXT", "Wert"=0}  # Rechnenbefehle
                # "Next"
                n82 = Build Array (concatenate)(w288, w287) -> (w289:T2[])
              }
              frame 76 {
                w291 = T2 {"Operation"=enum."Fertig", "Wert"=0}  # Rechnenbefehle
                # "Fertig"
                n83 = Build Array (concatenate)(w292, w291) -> (w293:T2[])
              }
            }
            n84 = Empty Array?(array=w197) -> (empty?=w196:bool)
          }
          "SA2 Operator" <- w180
          n85 = Bundle By Name(cluster=T1 {"Start Adress"=[0, 1], "Block Size"=[0, 6, 255, 240], "Checksum"=[]}, "Checksum"=w156, "Start Adress"=w162, "Block Size"=w161) -> (→"Download Parameter":T1)
        }
        frame Error {
        }
      }
    }
    frame Error {
    }
  }
  "error out" <- w2
